vi "Set Expected Channel Count.vi"(8 "error in":errorcluster, 11 "NI 9475 test in":refnum<class "NI 9475 Test.lvclass">) -> (0 "error out":errorcluster, 3 "NI 9475 test out":refnum<class "NI 9475 Test.lvclass">)   [LabVIEW 2020, in "NI 9475 Test.lvclass"]
uses:
  NI 9475 Test.lvclass
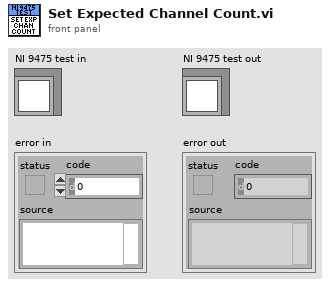
[diagram p1: front panel]
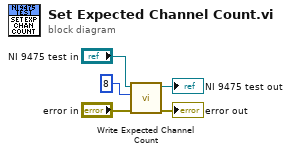
[diagram p0: block diagram]
diagram:
  n1 = call-dynamic "Write Expected Channel Count.vi"("error in"="error in", "expected channel count"=8, "module test in"="NI 9475 test in") -> ("error out"=→"error out":errorcluster, "module test out"=→"NI 9475 test out":refnum<class "NI 9475 Test.lvclass">)  [unwired: 7 in]
